vi "Write and Read XML File.vi"() -> ()   [LabVIEW 2011]
panel:
  out "Playlist read":T1
  in  "Delete File When Done (TRUE)":bool=TRUE
  out "XML File Path":path
  out "File Contents (for reference only)":string
  in  "Playlist to write":T1={"#attributes"={"Version"="1.0", "Creator"="LabVIEW"}, "Name"="Funky Grooves", "Song"=[{"Title"="Super Freak", "Artist"="Rick James"}, {"Title"="U Can't Touch This", "Artist"="MC Hammer"}, {"Title"="I Got You (I Feel Good)", "Artist"="James Brown"}, {"Title"="Get Down On It", "Artist"="Kool & The Gang"}]}
  # "Run this VI to write the 'Playlist' cluster (left) to an XML File and then read the data and format back into 'Playlist Out' cluster (right)"
  # "Contents to Write"
  # "Read Contents"
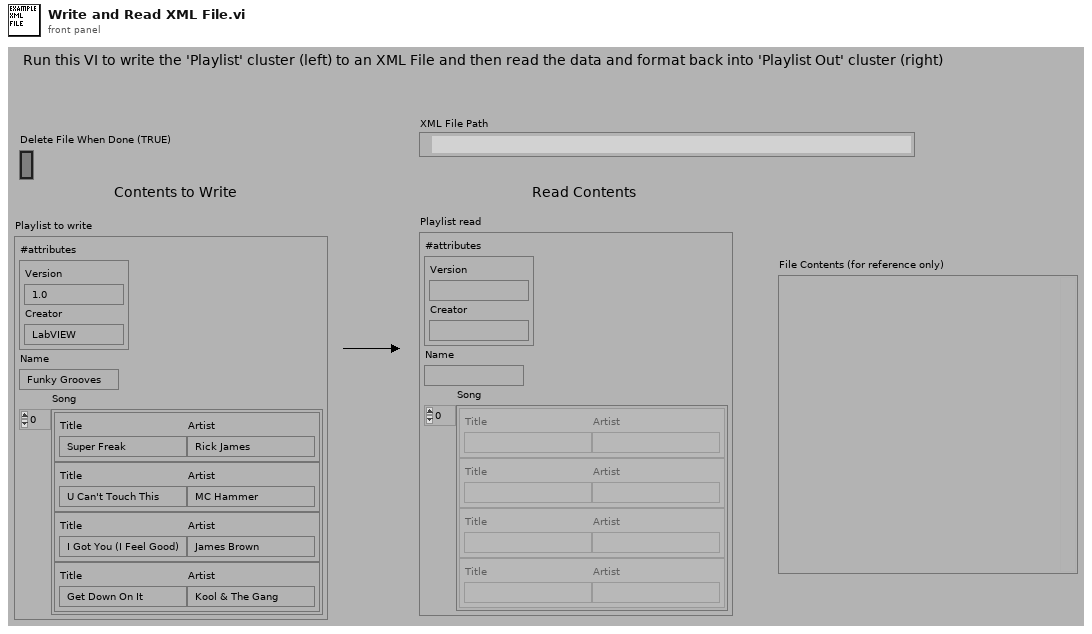
[diagram p1: front panel]
types:
  T1 = cluster{"#attributes":cluster{"Version":string, "Creator":string}, "Name":string, "Song":cluster{"Title":string, "Artist":string}[]}
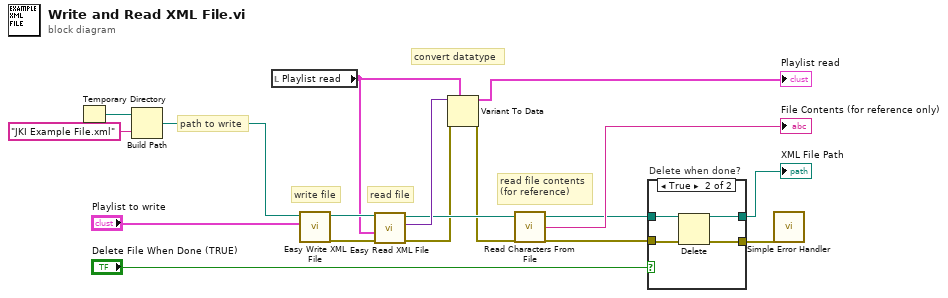
[diagram p0: block diagram]
diagram:
  # "convert datatype"
  # "path to write"
  # "read file contents\n(for reference)"
  # "read file"
  # "write file"
  n1 = Temporary Directory() -> (w17:path)
  n2 = Build Path(base path=w17, name or relative path="JKI Example File.xml") -> (appended path=w15:path)
  n3 = local read "Playlist read"() -> (w1:T1)
  n4 = call "Easy Write XML File.vi"("LabVIEW Data"="Playlist to write", "XML File Path"=w15) -> ("error out"=w13:errorcluster, "XML File Path (duplicate)"=w14:path)  [unwired: 8 in]
  n5 = call "Easy Read XML File.vi"("error in (no error)"=w13, "LabVIEW Data (Type)"=w1, "XML File Path"=w14) -> ("error out"=w4:errorcluster, "LabVIEW Data"=w12:variant, "XML File Path (duplicate)"=w10:path)  [unwired: 6 in]
  n6 = Variant To Data(error in=w4, type=w1, Variant=w12) -> (data=→"Playlist read":T1, error out=w3:errorcluster)
  n7 = call <vilib>:"Read Characters From File.vi"("file path (dialog if empty)"=w10) -> ("new file path (NotAPath if cancelled)"=w8:path, "character string"=→"File Contents (for reference only)":string)  [unwired: 5 in, 2 out]
  n8 = case "Delete when done?" shown="True" "Delete File When Done (TRUE)" {
    tunnel: w8 -> [w19 w23]
    tunnel: w3 -> [w18 w22]
    tunnel: [w18 w21] -> w7
    tunnel: [w19 w20] -> w5
    frame False {
    }
    frame True {
      n9 = Delete(path (use dialog)=w23, error in=w22) -> (deleted path=w20:path, error out=w21:errorcluster)  [unwired: 3 in, 1 out]
    }
  }
  "XML File Path" <- w5
  n10 = call <vilib>:"Simple Error Handler.vi"("error in (no error)"=w7) -> ()  [unwired: 4 in, 5 out]
